vi "WS1050_Ke2400_Single Voltage_Ver1.0.vi"(0 "Voltage P1":refnum<visa-resource-name>="GPIB0::5::INSTR", 5 "Input 1":dbl, 11 "error in (no error)":errorcluster) -> (2 "Voltage Output(V()":dbl, 4 "Voltage P1 Out":refnum<visa-resource-name>, 8 "Current 1":sgl, 15 "error out":errorcluster)   [LabVIEW 2012]
doc: "This VI configures the specifies power supply's channel to generate a DC voltage by taking the following steps:\n\n1) Configure current limit.\n\n2) Configure the over voltage protection.\n\n3) Configure the voltage level.\n\n4) Enable or disable the power output.\n\n5) Query the over voltage output state.\n\nNotes:\n\n(1) This VI takes a couple seconds to finish so that it may correctly get the current OVP value."
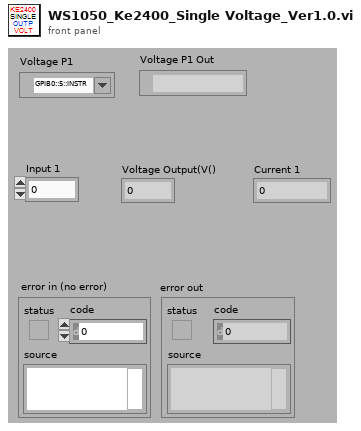
[diagram p1: front panel]
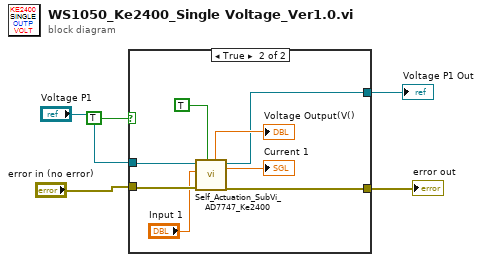
[diagram p0: block diagram]
diagram:
  n1 = case shown="True" TRUE {
    tunnel: [w7 w8] -> w2
    tunnel: "Voltage P1" -> [w6 w14]
    tunnel: "error in (no error)" -> [w7 w15]
    tunnel: [w6 w9] -> w1
    frame False {
    }
    frame True {
      n2 = call "Self_Actuation_SubVi_AD7747_Ke2400.vi"("Enable Output (T: Enable)"=TRUE, "error in (no error)"=w15, "Output Level (0)"="Input 1", "VISA resource name"=w14) -> ("error out"=w8:errorcluster, "Current"=→"Current 1":sgl, "VISA resource name out"=w9:refnum<visa-resource-name>, "Voltage Output(V()"=→"Voltage Output(V()":dbl)  [unwired: 4 in]
    }
  }
  "error out" <- w2
  "Voltage P1 Out" <- w1
